vi "gfitsio-read-image-subset-dbl-1d.vi"(4 "lpixel (-1: rest)":i32=-1, 6 "fpixel (1)":i32=1, 7 "inc (1)":i32=1, 8 "error in (no error)":errorcluster, 9 "nulval (0: don't check)":dbl, 11 "gfits refnum":T1) -> (0 "error out":errorcluster, 1 "anynul":bool, 2 "data":dbl[](array[numeric]), 3 "dup gfits refnum":T1)   [LabVIEW 2019, in "gfitsio.lvlib"]
doc: "Read a rectangular subimage (or the whole image) from the FITS data array. <B>fpixel</B> and <B>lpixel</B> give the coordinates of the first (lower left corner) and last (upper right corner) pixels to be read from the FITS image. Undefined FITS array elements will be set equal to <B>nullval</B> unless <B>nulval</B> is zero in which case no checks for undefined pixels will be performed."
uses:
  gfitsio.lvlib
  gfitsio-refnum.ctl
  cfitsio-hdutypes.ctl
  gfitsio.dll
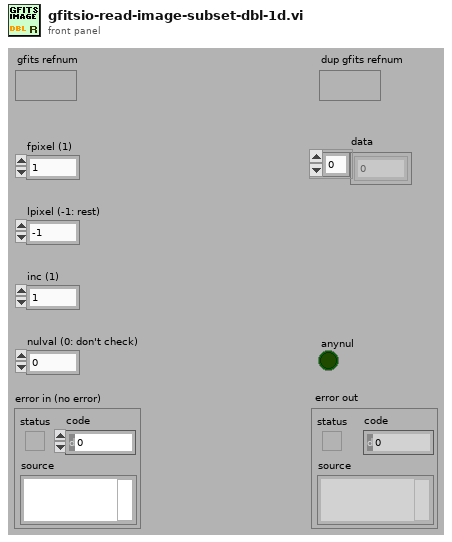
[diagram p1: front panel]
types:
  T1 = typedef "gfitsio.lvlib/gfitsio-refnum.ctl" = refnum<k1>
  T2 = typedef "gfitsio.lvlib/cfitsio-hdutypes.ctl" = i32
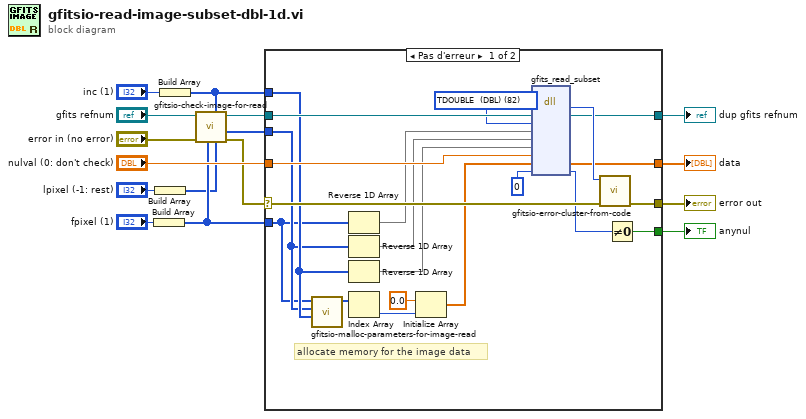
[diagram p0: block diagram]
diagram:
  n1 = Build Array("fpixel (1)") -> (w3:i32[])
  n2 = Build Array("lpixel (-1: rest)") -> (w2:i32[])
  n3 = Build Array("inc (1)") -> (w1:i32[])
  n4 = call "gfitsio-check-image-for-read.vi"("lpixel"=w2, "inc"=w1, "fpixel"=w3, "error in (no error)"="error in (no error)", "gfits refnum"="gfits refnum") -> ("error out"=w5:errorcluster, "lpixel out"=w4:i32[], "dup gfits refnum"=w10:T1)  [unwired: 4 in]
  n5 = case shown="Pas d'erreur" w5 {
    selector: w5 -> [w32 w38]
    tunnel: [w36 w38] -> w15
    tunnel: w10 -> [w34 w39]
    tunnel: [w33 w39] -> w16
    tunnel: "nulval (0: don't check)" -> [w31 _]
    tunnel: [w29 _] -> w13
    tunnel: [w28 _] -> w12
    tunnel: w3 -> [w21 _]
    tunnel: w4 -> [w22 _]
    tunnel: w1 -> [w23 _]
    frame No Error {
      w27 = T2 82 items=["TBIT"=1, "TBYTE  (U8)"=11, "TSBYTE  (I8)"=12, "TLOGICAL"=14, "TSTRING"=16, "TUSHORT  (U16)"=20, "TSHORT  (I16)"=21, "TUINT"=31, "TULONG  (U32)"=40, "TLONG  (I32)"=41, "TFLOAT  (SGL)"=42, "TLONGLONG  (I64)"=81, "TDOUBLE  (DBL)"=82, "TCOMPLEX  (CSG)"=83, "TDOUBLECOMPLEX  (CDB)"=163] ("cfitsio datatype")
      # "allocate memory for the image data"
      n6 = call "gfitsio-malloc-parameters-for-image-read.vi"("inc"=w23, "lpixel"=w22, "fpixel"=w21) -> ("image dimensions"=w18:i32[])  [unwired: 8 in]
      n7 = Reverse 1D Array(array=w21) -> (reversed array=w24:i32[])
      n8 = Reverse 1D Array(array=w22) -> (reversed array=w25:i32[])
      n9 = Reverse 1D Array(array=w23) -> (reversed array=w26:i32[])
      n10 = Index Array(array=w18) -> (element=w17:i32)  [unwired: 1 in]
      n11 = Initialize Array(0.0 ("element"), w17) -> (w19:dbl[])
      n12 = dll-call lib="C:/BonOMM_git/SubVIs/gfitsio/gfitsio.dll" fn="gfits_read_subset"("dup gfits refnum"=w34, "datatype"=w27, "fpixel"=w24, "lpixel"=w25, "inc"=w26, "nulval"=w31, "array"=w19, "anynul"=0) -> (w37:i32, "dup gfits refnum"=w33:T1, "array"=w28:dbl[], "anynul"=w30:i32)  [unwired: 8 in, 2 out]
      n13 = call "gfitsio-error-cluster-from-code.vi"("error in (no error)"=w32, "error code"=w37) -> ("error out"=w36:errorcluster)  [unwired: 9 in]
      n14 = Not Equal To 0?(x=w30) -> (x != 0?=w29:bool)
    }
    frame Error {
    }
  }
  "dup gfits refnum" <- w16
  "error out" <- w15
  "anynul" <- w13
  "data" <- w12
